vi "lv push doubles.vi"(8 "error in":errorcluster, 9 "values":dbl[](array[numeric]), 10 "timestamps (ns)":i64[](array[numeric]), 11 "channel handle":i32) -> (0 "error out":errorcluster)   [LabVIEW 2026]
uses:
  bin/nominalClient_64.dll
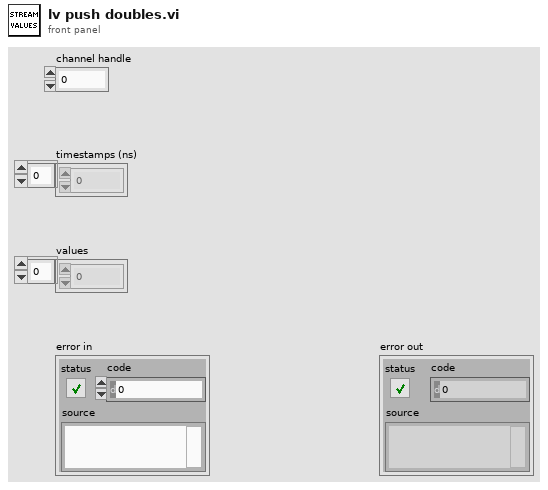
[diagram p1: front panel]
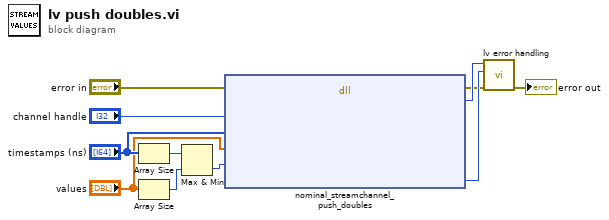
[diagram p0: block diagram]
diagram:
  n1 = Array Size(array="timestamps (ns)") -> (size(s)=w4:i32)
  n2 = Array Size(array="values") -> (size(s)=w5:i32)
  n3 = Max & Min(x=w4, y=w5) -> (min(x,y)=w6:i32)  [unwired: 1 out]
  n4 = dll-call lib="C:/sw/nominal-c/bin/nominalClient_64.dll" fn="nominal_streamchannel_push_doubles"(error in="error in", "channel"="channel handle", "timestamps ns"="timestamps (ns)", "data values"="values", "count"=w6) -> (error out=w7:errorcluster, "return type"=w9:i32, "errorout"=w10:i32)  [unwired: 7 in, 1 out]
  n5 = call "lv error handling.vi"("error in"=w7, "error handle"=w10, "return code"=w9) -> ("error out"=→"error out":errorcluster)  [unwired: 8 in]
